vi "SmartCursorTest.vi"() -> ()   [LabVIEW 2026]
uses:
  <vilib>/Utility/miscctls.llb/LVPoint32TypeDef.ctl
panel:
  out "appended array":T1[](array[typedef]) {"Horizontal" format="%#.2f"; "Vertical" format="%#.3f"}
  in  "Stop":bool
  out "Waveform Graph":dynamicdata(graph)
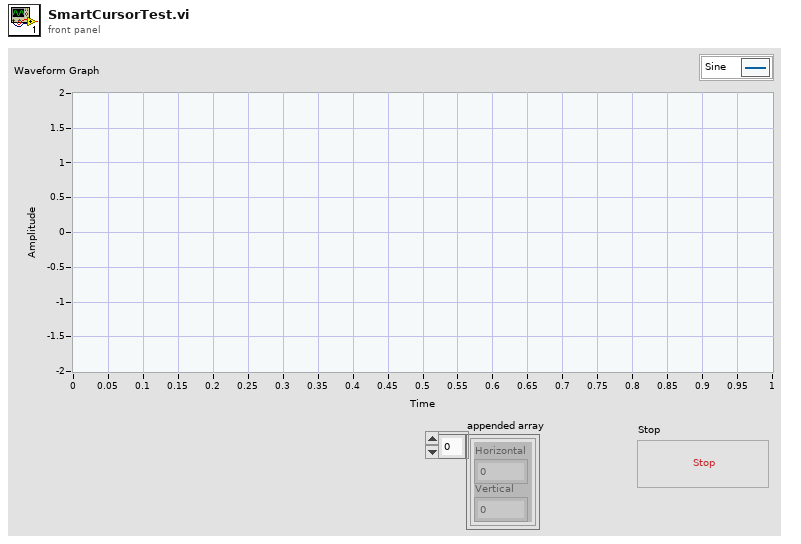
[diagram p1: front panel]
types:
  T1 = typedef "LVPoint32TypeDef.ctl" = cluster{"Horizontal":dbl, "Vertical":dbl}
  T2 = typedef "LVPoint32TypeDef.ctl" = cluster{"Horizontal":i32, "Vertical":i32}
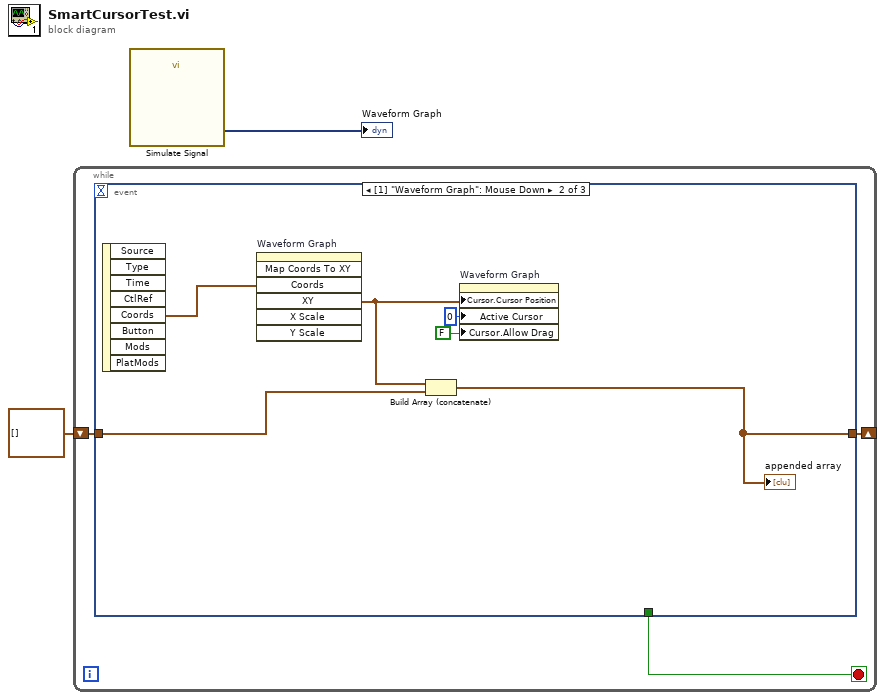
[diagram p0: block diagram]
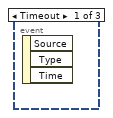
[diagram p2: hidden frame]
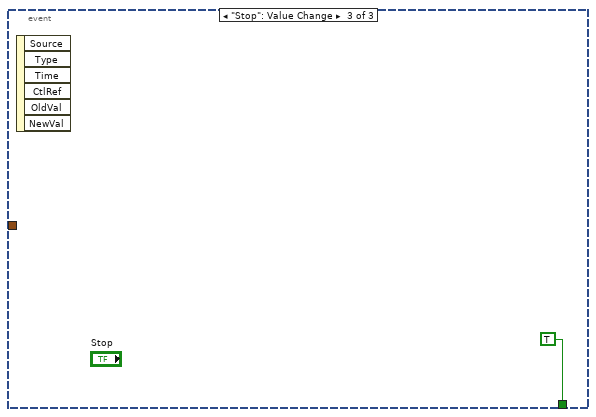
[diagram p3: hidden frame]
diagram:
  n1 = while {
    shift-right: [w3] -> _
    shift-left: T1[] [] -> [w4]
    stop <- w5 stop-if-true
    n2 = event shown="[1] \"Waveform Graph\": Mouse Down" {
      selector: _ -> [_ _ _]
      dyn-events: _ -> [_ _ _]
      timeout: _ -> [_ _ _]
      tunnel: [_ _ TRUE] -> w5
      tunnel: w4 -> [_ w10 _]
      tunnel: [_ w8 _] -> w3
      event Timeout {
        n3 = event-data() -> ()  [unwired: 1 in, 3 out]
      }
      event "Waveform Graph": Mouse Down {
        n4 = event-data() -> ("Coords"=w6:T2)  [unwired: 1 in, 7 out]
        n5 = invoke on="Waveform Graph" class="WFGraph (strict)" method="Map Coords To XY"("Coords"=w6) -> ("XY"=w11:cluster{"X":dbl, "Y":dbl})  [unwired: 6 in, 6 out]
        n6 = Build Array (concatenate)(w11, w10) -> (w8:T1[])
        "appended array" <- w8
        n7 = property on="Waveform Graph" class="WFGraph (strict)"("Cursor.Cursor Position"=w11, "Active Cursor"=u32 0, "Cursor.Allow Drag"=FALSE) -> ()  [unwired: 2 in, 2 out]
      }
      event "Stop": Value Change {
        n8 = event-data() -> ()  [unwired: 1 in, 6 out]
      }
    }
  }
  n9 = call "Simulate Signal"() -> ("Sine"=→"Waveform Graph":dynamicdata)  [unwired: 14 in, 1 out]
